vi "Configure Adjacent Channel Power (Offset Setup Advanced).vi"(0 "VISA resource name":refnum<visa-resource-name>, 5 "ACP Advanced Rolloff Rate":dbl[](array[numeric]) min=0.01 max=1.0, 7 "ACP Advanced Offset Filter":i32[](array[ring]) items=["Rect", "Nyquist", "Rnyquist"], 9 "ACP Advanced Offset Bandwidth":dbl[](array[numeric]) min=1.0 max=125000000.0, 11 "error in (no error)":errorcluster, 12 "ACP Advanced Offset":i32[](array[ring]) items=["Off", "On"]) -> (4 "VISA resource name out":refnum<visa-resource-name>, 15 "error out":errorcluster)   [LabVIEW 2020, in "Anritsu Signal Analyzer Series.lvlib"]
doc: "Configures the offset (Advanced Mode) for ACP measurement."
uses:
  Anritsu Signal Analyzer Series.lvlib
panel:
  # "Hz"
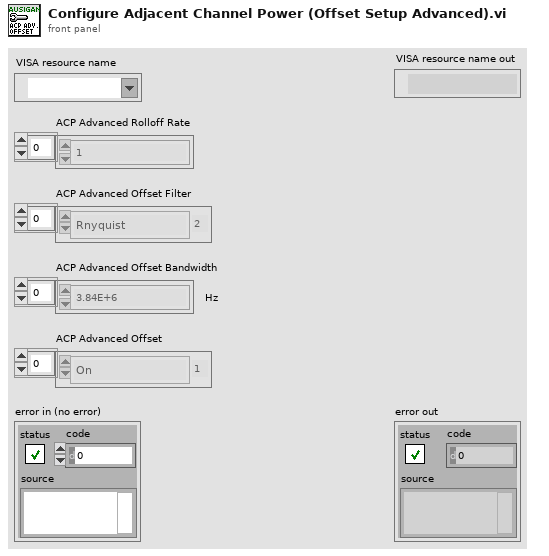
[diagram p1: front panel]
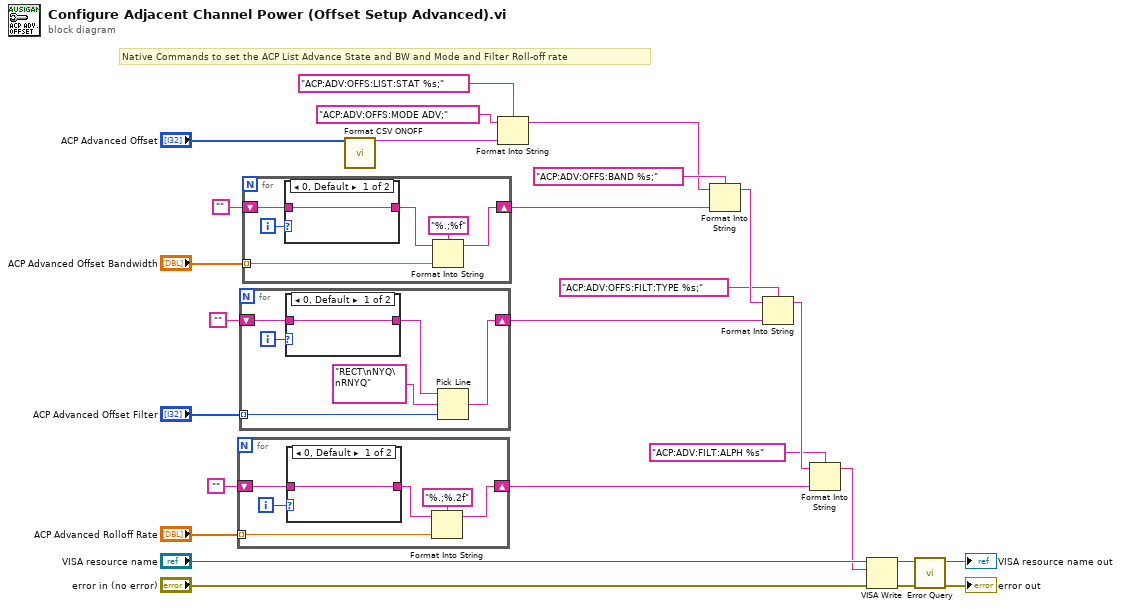
[diagram p0: block diagram]
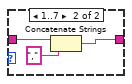
[diagram p2: hidden frame]
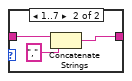
[diagram p3: hidden frame]
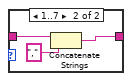
[diagram p4: hidden frame]
diagram:
  # "Native Commands to set the ACP List Advance State and BW and Mode and Filter Roll-off rate"
  n1 = for {
    shift-right: [w27] -> w10
    shift-left: "" -> [w31]
    tunnel: "ACP Advanced Rolloff Rate" -> [w29] mode=indexing
    i -> [w32]
    n2 = case shown="0, Default" w32 {
      tunnel: w31 -> [w33 w36]
      tunnel: [w33 w34] -> w28
      frame 0, Default {
      }
      frame 1..7 {
        n3 = Concatenate Strings(w36, "," ("string")) -> (w34:string)
      }
    }
    n4 = Format Into String(format string="%.;%.2f" ("_CommandSet"), initial string=w28, w29) -> (resulting string=w27:string)  [unwired: 1 in, 1 out]
  }
  n5 = for {
    shift-right: [w37] -> w14
    shift-left: "" -> [w41]
    tunnel: "ACP Advanced Offset Filter" -> [w39] mode=indexing
    i -> [w42]
    n6 = case shown="0, Default" w42 {
      tunnel: w41 -> [w43 w46]
      tunnel: [w43 w44] -> w38
      frame 0, Default {
      }
      frame 1..7 {
        n7 = Concatenate Strings(w46, "," ("string")) -> (w44:string)
      }
    }
    n8 = Pick Line(string ("")=w38, multi-line string="RECT\nNYQ\nRNYQ" ("複数行文字列"), line index=w39) -> (output string=w37:string)
  }
  n9 = for {
    tunnel: "ACP Advanced Offset Bandwidth" -> [w49] mode=indexing
    shift-right: [w47] -> w17
    shift-left: "" -> [w51]
    i -> [w52]
    n10 = case shown="0, Default" w52 {
      tunnel: w51 -> [w53 w56]
      tunnel: [w53 w54] -> w48
      frame 0, Default {
      }
      frame 1..7 {
        n11 = Concatenate Strings(w56, "," ("string")) -> (w54:string)
      }
    }
    n12 = Format Into String(format string="%.;%f" ("_CommandSet"), initial string=w48, w49) -> (resulting string=w47:string)  [unwired: 1 in, 1 out]
  }
  n13 = call "Format CSV ONOFF.vi"("Data_In"="ACP Advanced Offset") -> ("Data_out"=w1:string)  [unwired: 14 in]
  n14 = Format Into String(format string="ACP:ADV:OFFS:LIST:STAT %s;" ("_CommandSet"), initial string="ACP:ADV:OFFS:MODE ADV;" ("_CommandSet"), w1) -> (resulting string=w4:string)  [unwired: 1 in, 1 out]
  n15 = Format Into String(format string="ACP:ADV:OFFS:BAND %s;" ("_CommandSet"), initial string=w4, w17) -> (resulting string=w13:string)  [unwired: 1 in, 1 out]
  n16 = Format Into String(format string="ACP:ADV:OFFS:FILT:TYPE %s;" ("_CommandSet"), initial string=w13, w14) -> (resulting string=w9:string)  [unwired: 1 in, 1 out]
  n17 = Format Into String(format string="ACP:ADV:FILT:ALPH %s" ("_CommandSet"), initial string=w9, w10) -> (resulting string=w3:string)  [unwired: 1 in, 1 out]
  n18 = VISA Write(VISA resource name="VISA resource name", write buffer=w3, error in (no error)="error in (no error)") -> (VISA resource name out=w7:refnum<visa-resource-name>, error out=w6:errorcluster)  [unwired: 1 out]
  n19 = call "Error Query.vi"("error in (no error)"=w6, "VISA resource name"=w7) -> ("error out"=→"error out":errorcluster, "VISA resource name out"=→"VISA resource name out":refnum<visa-resource-name>)  [unwired: 6 in, 2 out]
